vi "All_Bundled_Resquest2.vi"(5 "Data":string) -> (2 "out_All_Request2":T1)   [LabVIEW 2021]
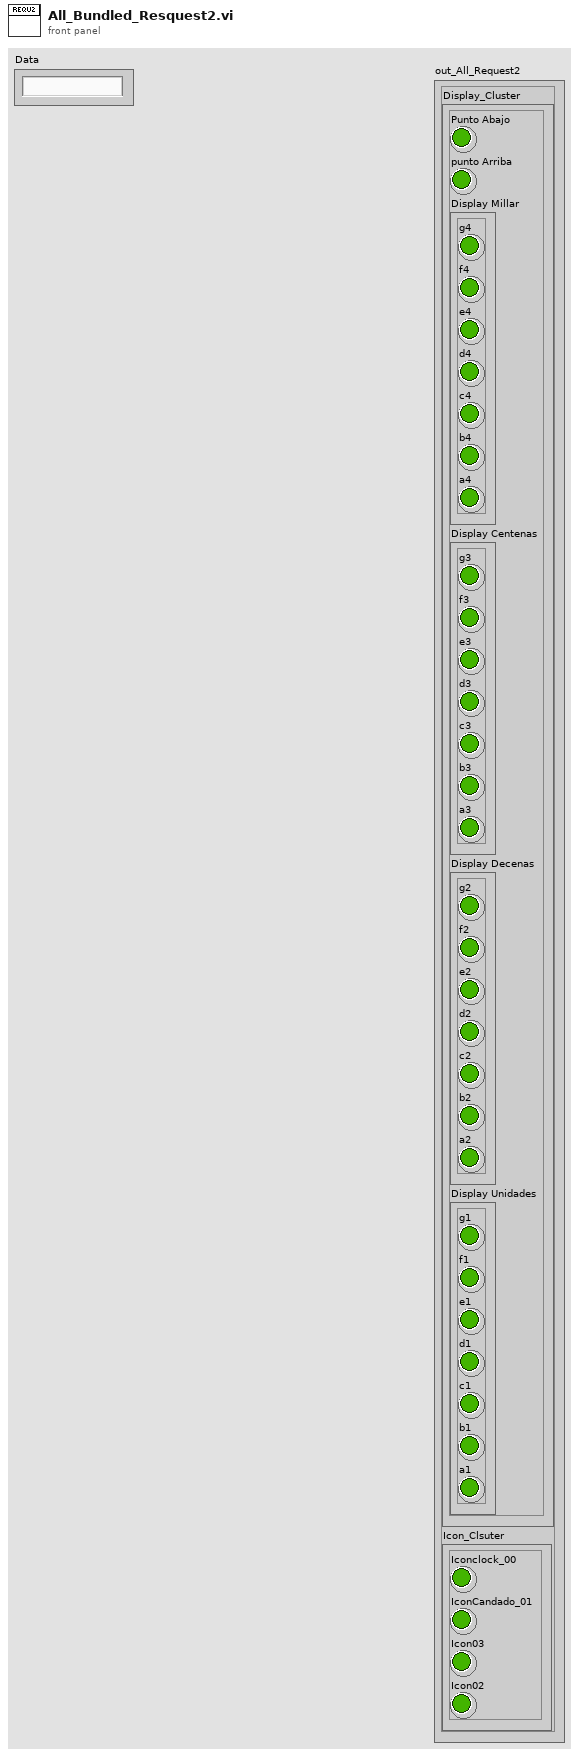
[diagram p1: front panel]
types:
  T1 = cluster{"Display_Cluster":cluster{"Punto Abajo":bool, "punto Arriba":bool, "Display Millar":cluster{"g4":bool, "f4":bool, "e4":bool, "d4":bool, "c4":bool, "b4":bool, "a4":bool}, "Display Centenas":cluster{"g3":bool, "f3":bool, "e3":bool, "d3":bool, "c3":bool, "b3":bool, "a3":bool}, "Display Decenas":cluster{"g2":bool, "f2":bool, "e2":bool, "d2":bool, "c2":bool, "b2":bool, "a2":bool}, "Display Unidades":cluster{"g1":bool, "f1":bool, "e1":bool, "d1":bool, "c1":bool, "b1":bool, "a1":bool}}, "Icon_Clsuter":cluster{"Iconclock_00":bool, "IconCandado_01":bool, "Icon03":bool, "Icon02":bool}}
  T2 = cluster{"Iconclock_00":bool, "IconCandado_01":bool, "Icon03":bool, "Icon02":bool}
  T3 = cluster{"Punto Abajo":bool, "punto Arriba":bool, "Display Millar":cluster{"g4":bool, "f4":bool, "e4":bool, "d4":bool, "c4":bool, "b4":bool, "a4":bool}, "Display Centenas":cluster{"g3":bool, "f3":bool, "e3":bool, "d3":bool, "c3":bool, "b3":bool, "a3":bool}, "Display Decenas":cluster{"g2":bool, "f2":bool, "e2":bool, "d2":bool, "c2":bool, "b2":bool, "a2":bool}, "Display Unidades":cluster{"g1":bool, "f1":bool, "e1":bool, "d1":bool, "c1":bool, "b1":bool, "a1":bool}}
  T4 = cluster{"bit 0":bool, "bit 1":bool, "bit 2":bool, "bit 3":bool, "bit 4":bool, "bit 5":bool, "bit 6":bool, "bit 7":bool}
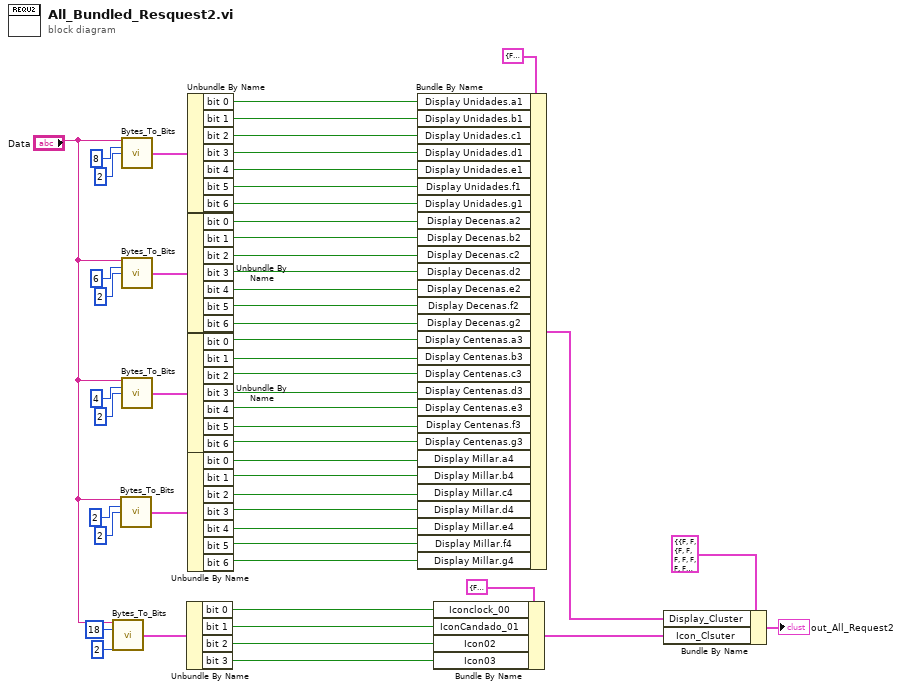
[diagram p0: block diagram]
diagram:
  n1 = call "Bytes_To_Bits.vi"("Data"="Data", "offset (0)"=18, "length (rest)"=2) -> ("output cluster"=w9:T4)  [unwired: 12 in]
  n2 = call "Bytes_To_Bits.vi"("Data"="Data", "offset (0)"=2, "length (rest)"=2) -> ("output cluster"=w23:T4)  [unwired: 12 in]
  n3 = call "Bytes_To_Bits.vi"("Data"="Data", "offset (0)"=8, "length (rest)"=2) -> ("output cluster"=w52:T4)  [unwired: 12 in]
  n4 = call "Bytes_To_Bits.vi"("Data"="Data", "offset (0)"=6, "length (rest)"=2) -> ("output cluster"=w43:T4)  [unwired: 12 in]
  n5 = call "Bytes_To_Bits.vi"("Data"="Data", "offset (0)"=4, "length (rest)"=2) -> ("output cluster"=w31:T4)  [unwired: 12 in]
  n6 = Unbundle By Name(w9) -> ("bit 0"=w8:bool, "bit 1"=w7:bool, "bit 2"=w6:bool, "bit 3"=w5:bool)
  n7 = Unbundle By Name(w52) -> ("bit 0"=w44:bool, "bit 1"=w45:bool, "bit 2"=w46:bool, "bit 3"=w47:bool, "bit 4"=w48:bool, "bit 5"=w49:bool, "bit 6"=w50:bool)
  n8 = Unbundle By Name(w43) -> ("bit 0"=w40:bool, "bit 1"=w39:bool, "bit 2"=w38:bool, "bit 3"=w37:bool, "bit 4"=w36:bool, "bit 5"=w35:bool, "bit 6"=w34:bool)
  n9 = Unbundle By Name(w31) -> ("bit 0"=w24:bool, "bit 1"=w25:bool, "bit 2"=w26:bool, "bit 3"=w27:bool, "bit 4"=w28:bool, "bit 5"=w29:bool, "bit 6"=w30:bool)
  n10 = Unbundle By Name(w23) -> ("bit 0"=w19:bool, "bit 1"=w18:bool, "bit 2"=w17:bool, "bit 3"=w16:bool, "bit 4"=w15:bool, "bit 5"=w14:bool, "bit 6"=w20:bool)
  n11 = Bundle By Name(cluster=T3 {"Punto Abajo"=FALSE, "punto Arriba"=FALSE, "Display Millar"={"g4"=FALSE, "f4"=FALSE, "e4"=FALSE, "d4"=FALSE, "c4"=FALSE, "b4"=FALSE, "a4"=FALSE}, "Display Centenas"={"g3"=FALSE, "f3"=FALSE, "e3"=FALSE, "d3"=FALSE, "c3"=FALSE, "b3"=FALSE, "a3"=FALSE}, "Display Decenas"={"g2"=FALSE, "f2"=FALSE, "e2"=FALSE, "d2"=FALSE, "c2"=FALSE, "b2"=FALSE, "a2"=FALSE}, "Display Unidades"={"g1"=FALSE, "f1"=FALSE, "e1"=FALSE, "d1"=FALSE, "c1"=FALSE, "b1"=FALSE, "a1"=FALSE}} ("Display cluster"), "Display Unidades.a1"=w44, "Display Unidades.b1"=w45, "Display Unidades.c1"=w46, "Display Unidades.d1"=w47, "Display Unidades.e1"=w48, "Display Unidades.f1"=w49, "Display Unidades.g1"=w50, "Display Decenas.a2"=w40, "Display Decenas.b2"=w39, "Display Decenas.c2"=w38, "Display Decenas.d2"=w37, "Display Decenas.e2"=w36, "Display Decenas.f2"=w35, "Display Decenas.g2"=w34, "Display Centenas.a3"=w24, "Display Centenas.b3"=w25, "Display Centenas.c3"=w26, "Display Centenas.d3"=w27, "Display Centenas.e3"=w28, "Display Centenas.f3"=w29, "Display Centenas.g3"=w30, "Display Millar.a4"=w19, "Display Millar.b4"=w18, "Display Millar.c4"=w17, "Display Millar.d4"=w16, "Display Millar.e4"=w15, "Display Millar.f4"=w14, "Display Millar.g4"=w20) -> (w2:T3)
  n12 = Bundle By Name(cluster=T2 {"Iconclock_00"=FALSE, "IconCandado_01"=FALSE, "Icon03"=FALSE, "Icon02"=FALSE} ("Cluster Icons"), "Iconclock_00"=w8, "IconCandado_01"=w7, "Icon02"=w6, "Icon03"=w5) -> (w3:T2)
  n13 = Bundle By Name(cluster=T1 {"Display_Cluster"={"Punto Abajo"=FALSE, "punto Arriba"=FALSE, "Display Millar"={"g4"=FALSE, "f4"=FALSE, "e4"=FALSE, "d4"=FALSE, "c4"=FALSE, "b4"=FALSE, "a4"=FALSE}, "Display Centenas"={"g3"=FALSE, "f3"=FALSE, "e3"=FALSE, "d3"=FALSE, "c3"=FALSE, "b3"=FALSE, "a3"=FALSE}, "Display Decenas"={"g2"=FALSE, "f2"=FALSE, "e2"=FALSE, "d2"=FALSE, "c2"=FALSE, "b2"=FALSE, "a2"=FALSE}, "Display Unidades"={"g1"=FALSE, "f1"=FALSE, "e1"=FALSE, "d1"=FALSE, "c1"=FALSE, "b1"=FALSE, "a1"=FALSE}}, "Icon_Clsuter"={"Iconclock_00"=FALSE, "IconCandado_01"=FALSE, "Icon03"=FALSE, "Icon02"=FALSE}}, "Display_Cluster"=w2, "Icon_Clsuter"=w3) -> (→"out_All_Request2":T1)
